vi "Configure Auto Port Extension.vi"(6 "Standard (1: Short)":i32(ring)=1 items=["Open", "Short"], 7 "Enable Auto Port Extension (T: Enable)":bool=TRUE, 8 "error in (no error)":errorcluster, 9 "Port ( 1)":i32=1, 10 "Channel (1)":i32=1, 11 "VISA resource name":refnum<visa-resource-name>) -> (0 "error out":errorcluster, 3 "VISA resource name out":refnum<visa-resource-name>)   [LabVIEW 2022 SP3, in "Agilent ENA Series.lvlib"]
doc: "Configures the auto port extension settings.\n\n<B>Note:</B> This VI is only valid for E5061B and E5070/5071B."
uses:
  <instrlib>/Agilent ENA Series/Agilent ENA Series.lvlib
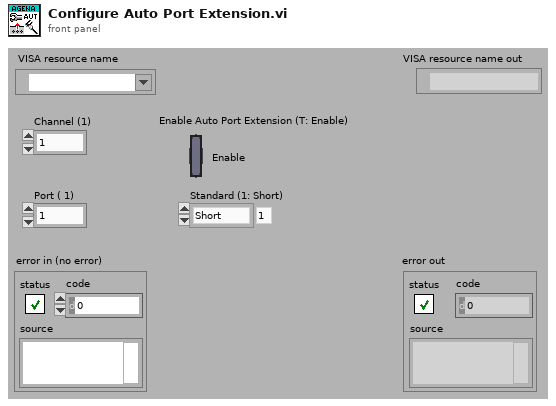
[diagram p1: front panel]
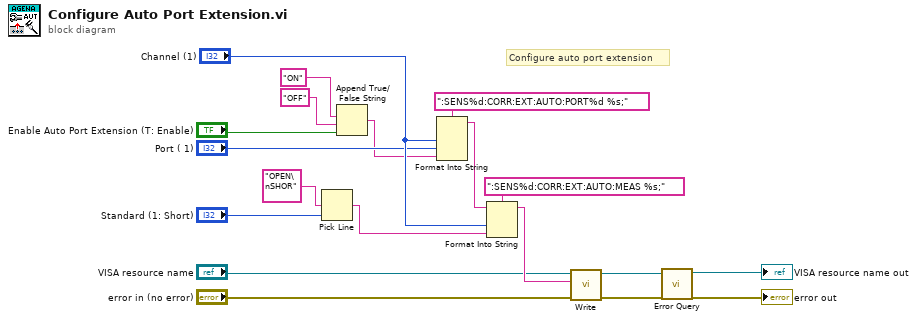
[diagram p0: block diagram]
diagram:
  # "Configure auto port extension"
  n1 = Pick Line(multi-line string="OPEN\nSHOR", line index="Standard (1: Short)") -> (output string=w8:string)  [unwired: 1 out]
  n2 = Append True/False String(1:"Enable Auto Port Extension (T: Enable)", 2:"OFF", 3:"ON") -> (0:w13:string)  [unwired: 1 out]
  n3 = Format Into String(format string=":SENS%d:CORR:EXT:AUTO:PORT%d %s;", "Channel (1)", "Port ( 1)", w13) -> (resulting string=w10:string)  [unwired: 2 in, 1 out]
  n4 = Format Into String(format string=":SENS%d:CORR:EXT:AUTO:MEAS %s;", initial string=w10, "Channel (1)", w8) -> (resulting string=w5:string)  [unwired: 1 in, 1 out]
  n5 = call <instrlib>:"Write.vi"("error in (no error)"="error in (no error)", "String ()"=w5, "VISA resource name"="VISA resource name") -> ("error out"=w1:errorcluster, "VISA resource name out"=w2:refnum<visa-resource-name>)  [unwired: 6 in, 1 out]
  n6 = call <instrlib>:"Error Query.vi"("error in (no error)"=w1, "VISA resource name"=w2) -> ("error out"=→"error out":errorcluster, "VISA resource name out"=→"VISA resource name out":refnum<visa-resource-name>)  [unwired: 8 out]
